vi "Error Query.vi"(8 "error in (no error)":errorcluster, 11 "VISA resource name":refnum<visa-resource-name>) -> (0 "error out":errorcluster, 1 "Error Message":string, 2 "Error Code":i32[](array[numeric]), 3 "VISA resource name out":refnum<visa-resource-name>)   [LabVIEW 2015, in "BK Precision 983X Series.lvlib"]
doc: "Queries the instrument for any errors in the instrument's error queue. It will continue to read errors until all errors have been read from the instrument. Any errors will be returned in the <B>error out</B> control.\n\n<B>Note:</B>\nThis VI is called automatically by most driver VIs so it is not usually necessary to call this in an application."
uses:
  <instrlib>/BK Precision 983X Series/BK Precision 983X Series.lvlib
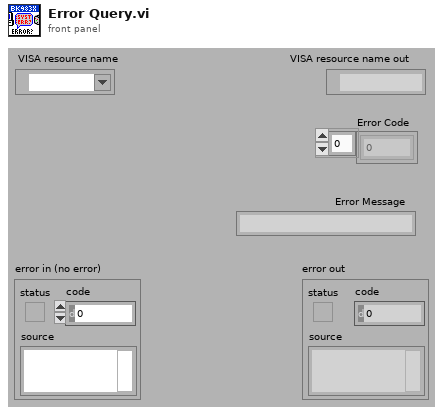
[diagram p1: front panel]
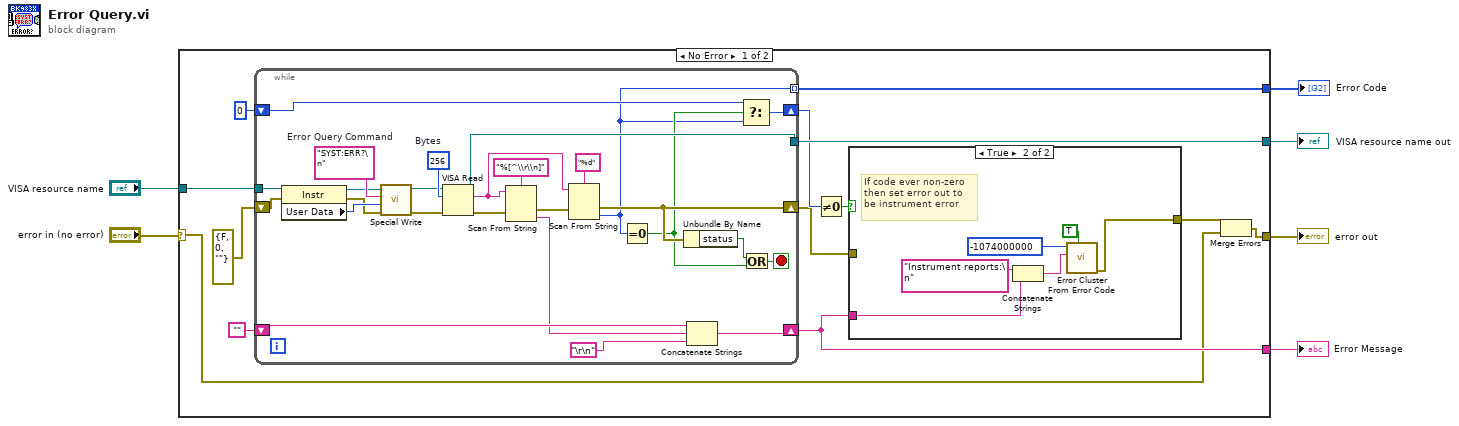
[diagram p0: block diagram]
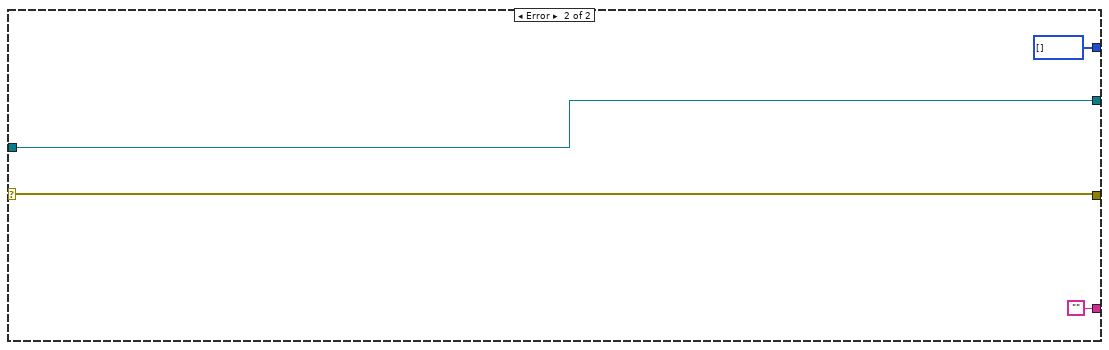
[diagram p3: hidden frame]
diagram:
  n1 = case shown="No Error" "error in (no error)" {
    selector: "error in (no error)" -> [w7 w53]
    tunnel: [w19 w56] -> w6
    tunnel: "VISA resource name" -> [w18 w56]
    tunnel: [w16 w53] -> w5
    tunnel: [w11 ""] -> w4
    tunnel: [w10 i32[] []] -> w3
    frame No Error {
      n2 = while {
        tunnel: [w52] -> w19
        tunnel: w18 -> [w37]
        shift-right: [w47] -> w11
        shift-left: "" -> [w31]
        shift-right: [w45] -> w12
        shift-left: 0 -> [w46]
        shift-right: [w44] -> w9
        shift-left: errorcluster {"status"=FALSE, "code"=0, "source"=""} ("error in (no error)") -> [w36]
        tunnel: [w41] -> w10 mode=indexing
        stop <- w49 stop-if-true
        w51 = u32 256  # Bytes
        w38 = "SYST:ERR?\n"  # Error Query Command
        n3 = property class="Instr"(reference=w37, error in=w36) -> (reference out=w33:refnum<visa-resource-name>, error out=w34:errorcluster, "User Data"=w35:u32)
        n4 = call <instrlib>:"Special Write.vi"("error in (no error)"=w34, "Delay (0 ms)"=w35, "Input String"=w38, "VISA resource name"=w33) -> ("error out"=w39:errorcluster, "VISA resource name out"=w40:refnum<visa-resource-name>)  [unwired: 6 in]
        n5 = VISA Read(VISA resource name=w40, byte count=w51, error in (no error)=w39) -> (VISA resource name out=w52:refnum<visa-resource-name>, read buffer=w27:string, error out=w29:errorcluster)  [unwired: 1 out]
        n6 = Scan From String(format string="%[^\\r\\n]", input string=w27, error in=w29) -> (error out=w28:errorcluster, output 1=w30:string)  [unwired: 2 in, 2 out]
        n7 = Scan From String(format string="%d", input string=w27, error in=w28) -> (error out=w44:errorcluster, output 1=w41:i32)  [unwired: 2 in, 2 out]
        n8 = Equal To 0?(x=w41) -> (x = 0?=w42:bool)
        n9 = Unbundle By Name(w44) -> ("status"=w43:bool)
        n10 = Concatenate Strings(w31, w30, "\r\n") -> (w47:string)
        n11 = Select(t=w46, s=w42, f=w41) -> (s? t:f=w45:i32)
        n12 = Or(x=w43, y=w42) -> (x .or. y?=w49:bool)
      }
      n13 = Not Equal To 0?(x=w12) -> (x != 0?=w14:bool)
      n14 = case shown="True" w14 {
        tunnel: w11 -> [_ w25]
        tunnel: [w20 w21] -> w13
        tunnel: w9 -> [w20 _]
        frame False {
        }
        frame True {
          # "If code ever non-zero\nthen set error out to\nbe instrument error"
          n15 = Concatenate Strings("Instrument reports:\n" ("Source"), w25) -> (w22:string)
          n16 = call <vilib>:"Error Cluster From Error Code.vi"("show call chain? (False)"=TRUE, "error message (\"\")"=w22, "error code (0)"=-1074000000 ("Code")) -> ("error out"=w21:errorcluster)  [unwired: 6 in]
        }
      }
      n17 = Merge Errors(w13, w7) -> (w16:errorcluster)
    }
    frame Error {
    }
  }
  "VISA resource name out" <- w6
  "error out" <- w5
  "Error Message" <- w4
  "Error Code" <- w3
